vi "Snake Check on Field.vi"(8 "error in (no error)":errorcluster, 10 "Bounds":T1, 11 "Snake in":refnum<class "Snake.lvclass">) -> (0 "error out":errorcluster, 2 "On Field?":bool, 3 "Snake out":refnum<class "Snake.lvclass">)   [LabVIEW 2020, in "Snake.lvclass"]
uses:
  Snake.lvclass
  Snake.lvclass/Snake.ctl
  d5d5b7fe-fb04-443c-ab60-a59b61c61f01.vi
  <vilib>/Comparison/Equal/Equal Functor/Equal Functor.lvclass
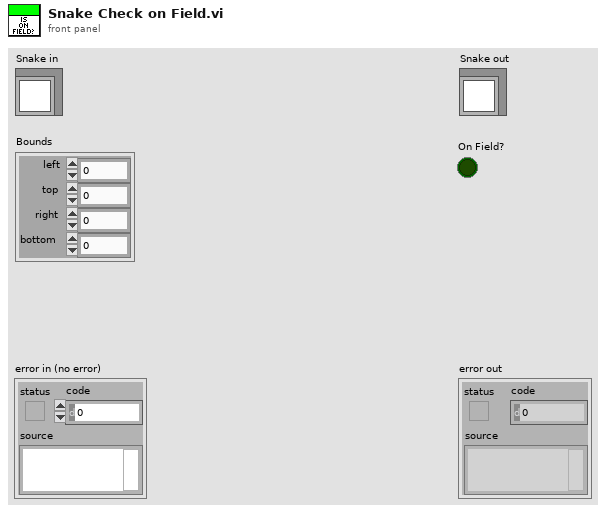
[diagram p1: front panel]
types:
  T1 = cluster{"left":u32, "top":u32, "right":u32, "bottom":u32}
  T2 = typedef "Snake.lvclass/Snake Segment STYP.ctl" = cluster{"Location":cluster{"x":u32, "y":u32}, "Direction":T3}
  T3 = typedef "Direction STYP.ctl" = enum16{"Up", "Down", "Left", "Right"}
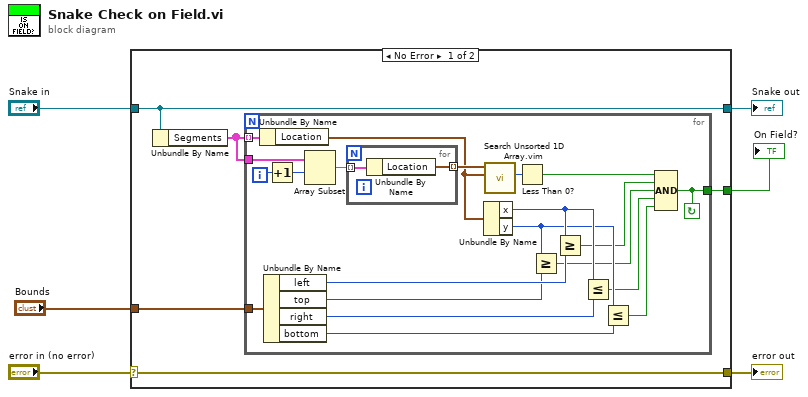
[diagram p0: block diagram]
diagram:
  n1 = case shown="No Error" "error in (no error)" {
    selector: "error in (no error)" -> [w11 w36]
    tunnel: [w11 w36] -> w5
    tunnel: [w10 w35] -> w3
    tunnel: "Snake in" -> [w10 w35]
    tunnel: "Bounds" -> [w8 _]
    tunnel: [w7 _] -> w1
    frame No Error {
      n2 = Unbundle By Name(w10) -> ("Segments"=w9:T2[])
      n3 = for {
        tunnel: w9 -> [w27] mode=indexing
        tunnel: w9 -> [w32]
        tunnel: w8 -> [w25]
        tunnel: [w12] -> w7
        i -> [w31]
        stop <- w12 continue-if-true
        n4 = Unbundle By Name(w27) -> ("Location"=w24:cluster{"x":u32, "y":u32})
        n5 = Unbundle By Name(w25) -> ("left"=w23:u32, "top"=w22:u32, "right"=w20:u32, "bottom"=w18:u32)
        n6 = Increment(x=w31) -> (x+1=w30:i32)
        n7 = Array Subset(array=w32, index=w30) -> (w29:T2[])  [unwired: 1 in]
        n8 = for {
          tunnel: w29 -> [w34] mode=indexing
          tunnel: [w33] -> w28 mode=indexing
          n9 = Unbundle By Name(w34) -> ("Location"=w33:cluster{"x":u32, "y":u32})
        }
        n10 = Unbundle By Name(w24) -> ("x"=w21:u32, "y"=w19:u32)
        n11 = call "Search Unsorted 1D Array.vim"("element"=w24, "unsorted 1D array"=w28) -> ("index of element"=w26:i32)  [unwired: 9 in]
        n12 = Less Than 0?(x=w26) -> (x < 0?=w17:bool)
        n13 = Greater Or Equal?(x=w19, y=w22) -> (x >= y?=w15:bool)
        n14 = Greater Or Equal?(x=w21, y=w23) -> (x >= y?=w16:bool)
        n15 = Less Or Equal?(x=w21, y=w20) -> (x <= y?=w14:bool)
        n16 = Less Or Equal?(x=w19, y=w18) -> (x <= y?=w13:bool)
        n17 = Compound Arithmetic op=AND(w17, w16, w15, w14, w13) -> (w12:bool)
      }
    }
    frame Error {
    }
  }
  "error out" <- w5
  "Snake out" <- w3
  "On Field?" <- w1
